vi "Configure Trigger.vi"(0 "VISA resource name":refnum<visa-resource-name>, 5 "Trigger Source (0: Immediate)":u16(ring) items=["Immediate", "Software (Bus)", "External"], 11 "error in (no error)":errorcluster, 12 "Auto Trigger Delay (T:Enable)":bool=TRUE, 13 "Manual Trigger Delay (0 s)":dbl) -> (4 "VISA resource name out":refnum<visa-resource-name>, 15 "error out":errorcluster)   [LabVIEW 2021, in "Agilent 34420.lvlib"]
doc: "Configures the trigger settings on the instrument.\n\n<B>Note:</B>\n\nUse this VI only with other low-level VIs. The high-level VIs automatically incorporate this functionality."
uses:
  <instrlib>/Agilent 34420/Agilent 34420.lvlib
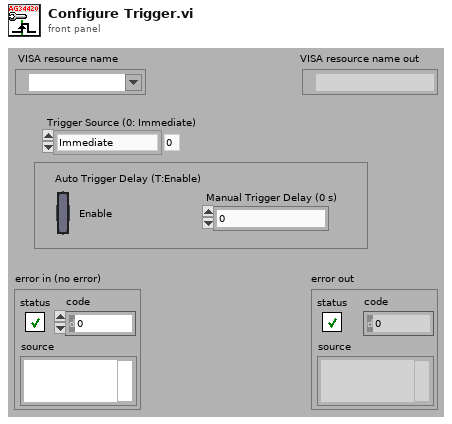
[diagram p1: front panel]
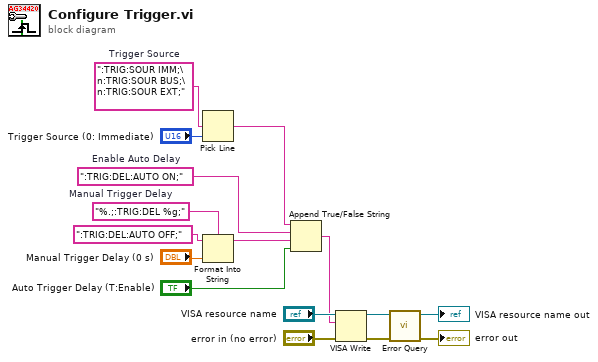
[diagram p0: block diagram]
diagram:
  w5 = ":TRIG:DEL:AUTO ON;"  # Enable Auto Delay
  w6 = "%.;:TRIG:DEL %g;"  # Manual Trigger Delay
  w13 = ":TRIG:SOUR IMM;\n:TRIG:SOUR BUS;\n:TRIG:SOUR EXT;"  # Trigger Source
  n1 = Pick Line(multi-line string=w13, line index="Trigger Source (0: Immediate)") -> (output string=w3:string)  [unwired: 1 in]
  n2 = Format Into String(format string=w6, initial string=":TRIG:DEL:AUTO OFF;", "Manual Trigger Delay (0 s)") -> (resulting string=w4:string)  [unwired: 1 in, 1 out]
  n3 = Append True/False String(1:"Auto Trigger Delay (T:Enable)", 2:w4, 3:w5, 4:w3) -> (0:w1:string)
  n4 = VISA Write(VISA resource name="VISA resource name", write buffer=w1, error in (no error)="error in (no error)") -> (VISA resource name out=w10:refnum<visa-resource-name>, error out=w9:errorcluster)  [unwired: 1 out]
  n5 = call <instrlib>:"Error Query.vi"("error in (no error)"=w9, "VISA resource name"=w10) -> ("error out"=→"error out":errorcluster, "VISA resource name out"=→"VISA resource name out":refnum<visa-resource-name>)  [unwired: 6 in, 2 out]
